vi "DNP3_Master_Station_Main.vi"() -> ()   [LabVIEW 2016, in "DNP3_Master_Station_Template.lvlib"]
uses:
  DNP3_Master_Station_Template.lvlib
  <vilib>/DNP3/DNP3_Master/Operation Mode.ctl
  <vilib>/DNP3/DNP3_Master/Poll Binary Input Variation.ctl
  <vilib>/DNP3/DNP3_Master/Analog Variation.ctl
  <vilib>/DNP3/DNP3_Master/Poll Analog Input Variation.ctl
  <vilib>/DNP3/DNP3_Master/Response Type.ctl
  SubVIs/Global_Bin_Out_Mode.vi
  SubVIs/Global_Bin_In_Var.vi
  SubVIs/Global_An_Out_Var.vi
  SubVIs/Global_An_Out_Mode.vi
  SubVIs/Global_An_In_Var.vi
  <vilib>/DNP3/DNP3_Master.lvlib
panel:
  out "POLL OS IND":bool=TRUE
  out "ENABLE MS IND":bool=TRUE
  out "RESET MS IND":bool
  out "STOP IND":bool
  in  "STOP":bool
  in  "MS Presets":T1(tab)
  in  "Disable Binary TX/RX":bool
  in  "LC1_MS_DNP3_Settings":T6={"Binary Out Mode"=6, "Binary In Variation"=0, "Analog Out Variation"=4, "Analog Out Mode"=6, "Analog In Variation"=0} {"Analog In Variation" items=["Default", "32-bit with Flag", "16-bit with Flag", "32-bit without Flag", "16-bit without Flag", "Single-prec with Flag", "Double-prec with Flag"]; "Analog Out Mode" items=["SBO"=0, "Select"=3, "Operate"=4, "Direct"=5, "Direct No Ack"=6]; "Analog Out Variation" items=["32-bit"=1, "16-bit"=2, "Single-prec"=3, "Double-prec"=4]; "Binary In Variation" items=["Default", "Packed Format", "With Flags"]; "Binary Out Mode" items=["SBO"=0, "Select"=3, "Operate"=4, "Direct"=5, "Direct No Ack"=6]}
  in  "LC1_MS_Network_Settings":T7={"Outstation IP"="10.158.130.104", "DNP3 Port"=20000, "DNP3 Master Address"=30026, "DNP3 Outstation Address"=30024}
  in  "LC1_MS_Network_Settings 2":T7
  in  "LC1_MS_DNP3_Settings 2":T6={"Binary Out Mode"=6, "Binary In Variation"=0, "Analog Out Variation"=4, "Analog Out Mode"=6, "Analog In Variation"=6} {"Analog In Variation" items=["Default", "32-bit with Flag", "16-bit with Flag", "32-bit without Flag", "16-bit without Flag", "Single-prec with Flag", "Double-prec with Flag"]; "Analog Out Mode" items=["SBO"=0, "Select"=3, "Operate"=4, "Direct"=5, "Direct No Ack"=6]; "Analog Out Variation" items=["32-bit"=1, "16-bit"=2, "Single-prec"=3, "Double-prec"=4]; "Binary In Variation" items=["Default", "Packed Format", "With Flags"]; "Binary Out Mode" items=["SBO"=0, "Select"=3, "Operate"=4, "Direct"=5, "Direct No Ack"=6]}
  in  "Disable Binary TX/RX 2":bool
  in  "LC1_MS_Network_Settings 3":T7
  in  "Disable Binary TX/RX 3":bool
  in  "LC1_MS_DNP3_Settings 3":T6={"Binary Out Mode"=6, "Binary In Variation"=0, "Analog Out Variation"=4, "Analog Out Mode"=6, "Analog In Variation"=6} {"Analog In Variation" items=["Default", "32-bit with Flag", "16-bit with Flag", "32-bit without Flag", "16-bit without Flag", "Single-prec with Flag", "Double-prec with Flag"]; "Analog Out Mode" items=["SBO"=0, "Select"=3, "Operate"=4, "Direct"=5, "Direct No Ack"=6]; "Analog Out Variation" items=["32-bit"=1, "16-bit"=2, "Single-prec"=3, "Double-prec"=4]; "Binary In Variation" items=["Default", "Packed Format", "With Flags"]; "Binary Out Mode" items=["SBO"=0, "Select"=3, "Operate"=4, "Direct"=5, "Direct No Ack"=6]}
  out "LC1_MS_RX_Status_Analog":T8=enum."Timeout"
  out "LC1_MS_RX_Status_Binary":T8=enum."Timeout"
  out "LC1_MS_TX_Status_Analog":T8=enum."Success"
  out "LC1_MS_TX_Status_Binary":T8=enum."Cancel"
  out "Main VI Iterations":i32=392
  out "MS SETTINGS CHANGED":bool
  in  "RESET MS":bool caption="Reset Outstation"
  in  "ENABLE MS":bool=TRUE
  in  "POLL OS":bool=TRUE
  out "MS SubVI Iterations":i32=64
  # "Settings Changed; Reset to Update"
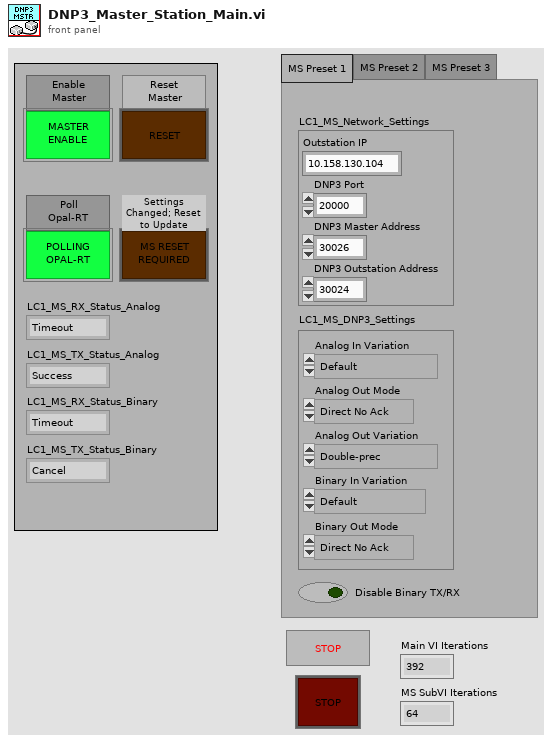
[diagram p1: front panel]
types:
  T1 = enum32{"MS Preset 1", "MS Preset 2", "MS Preset 3"}
  T2 = typedef "DNP3_Master.lvlib/Operation Mode.ctl" = u8
  T3 = typedef "DNP3_Master.lvlib/Poll Binary Input Variation.ctl" = u8
  T4 = typedef "DNP3_Master.lvlib/Analog Variation.ctl" = u8
  T5 = typedef "DNP3_Master.lvlib/Poll Analog Input Variation.ctl" = u8
  T6 = cluster{"Binary Out Mode":T2, "Binary In Variation":T3, "Analog Out Variation":T4, "Analog Out Mode":T2, "Analog In Variation":T5}
  T7 = cluster{"Outstation IP":string, "DNP3 Port":u16, "DNP3 Master Address":u16, "DNP3 Outstation Address":u16}
  T8 = typedef "DNP3_Master.lvlib/Response Type.ctl" = enum16{"Idle", "Buffering", "Pending", "Success", "Failure", "Mismatch", "Status Code", "IIN", "Timeout", "Cancel"}
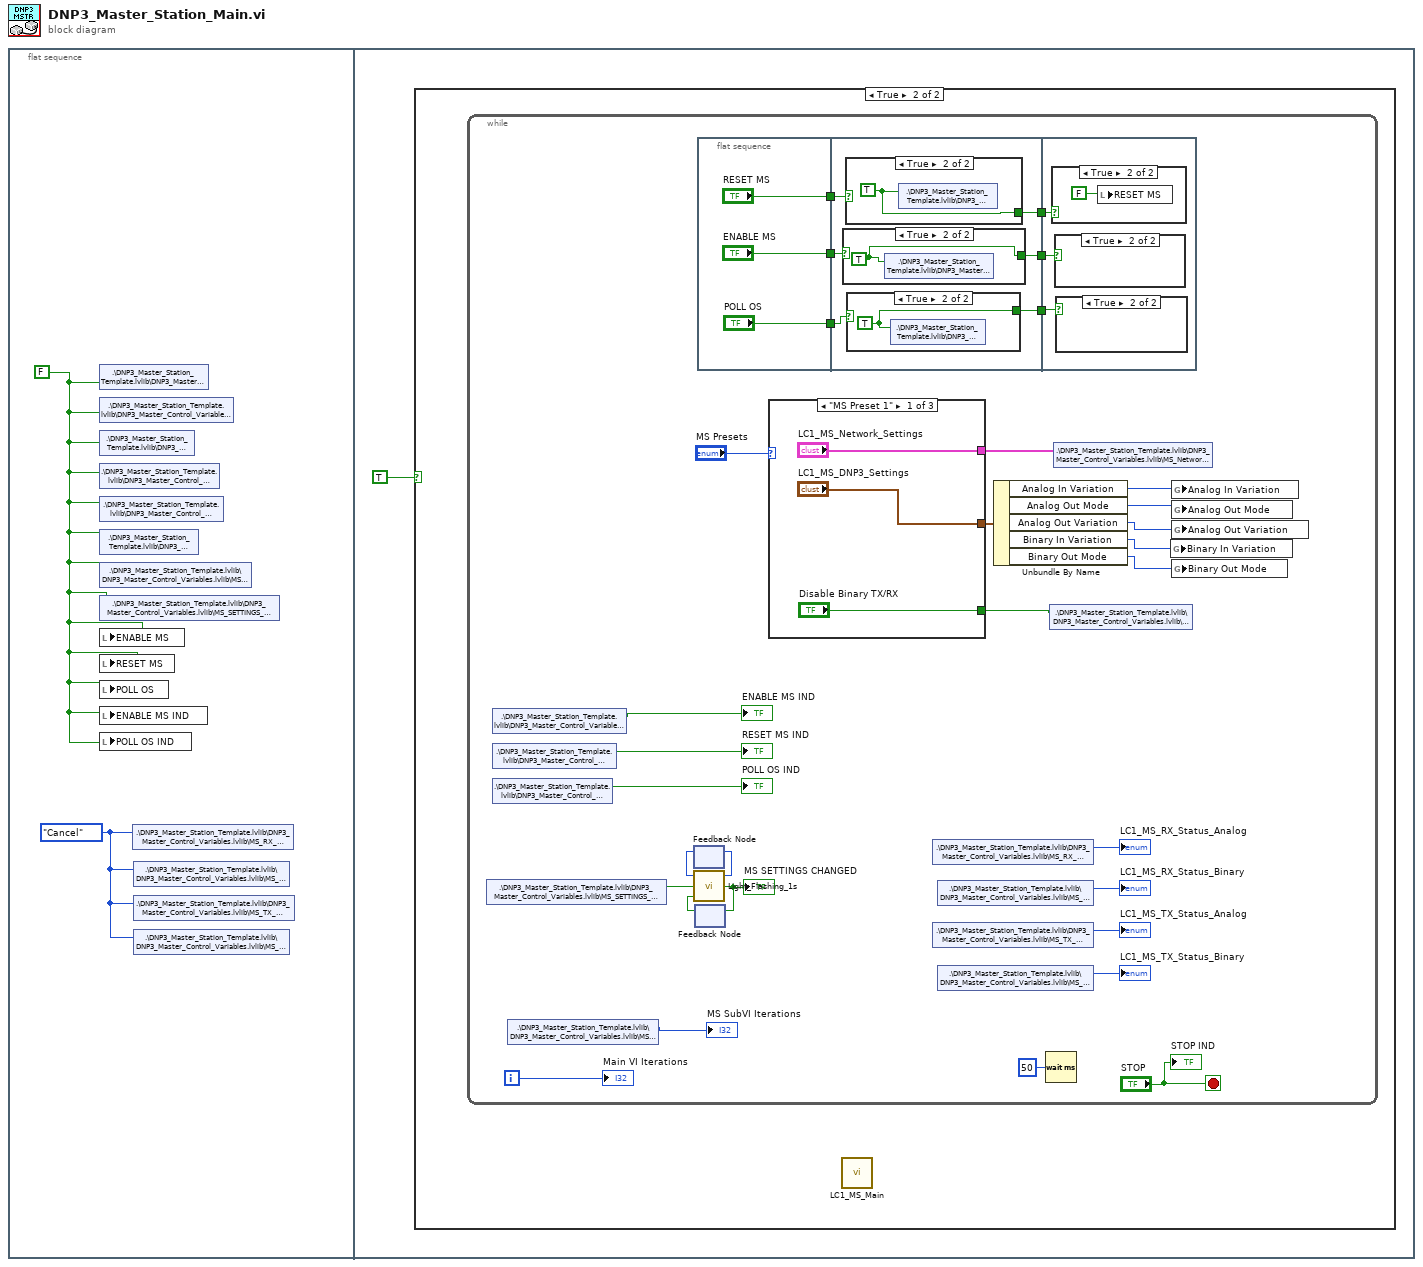
[diagram p0: block diagram]
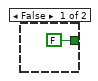
[diagram p3: hidden frame]
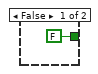
[diagram p4: hidden frame]
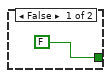
[diagram p5: hidden frame]
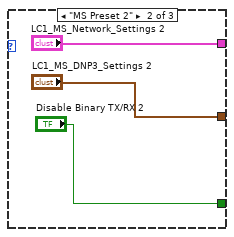
[diagram p9: hidden frame]
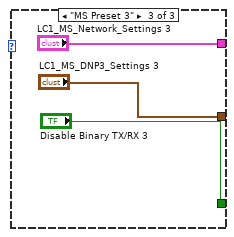
[diagram p10: hidden frame]
diagram:
  n1 = flat-sequence {
    frame #0 {
      w1 = Response_Type."Cancel" ("LC1_MS_RX_Status_Analog")
      w2 = FALSE ("LC1_MS_Enable")
      n2 = shared-variable ".\\DNP3_Master_Station_Template.lvlib\\DNP3_Master_Control_Variables.lvlib\\MS_ENABLE"(w2) -> ()  [unwired: 1 in, 1 out]
      n3 = shared-variable ".\\DNP3_Master_Station_Template.lvlib\\DNP3_Master_Control_Variables.lvlib\\MS_ENABLE_IND"(w2) -> ()  [unwired: 1 in, 1 out]
      n4 = shared-variable ".\\DNP3_Master_Station_Template.lvlib\\DNP3_Master_Control_Variables.lvlib\\MS_POLL"(w2) -> ()  [unwired: 1 in, 1 out]
      n5 = shared-variable ".\\DNP3_Master_Station_Template.lvlib\\DNP3_Master_Control_Variables.lvlib\\MS_POLL_IND"(w2) -> ()  [unwired: 1 in, 1 out]
      n6 = shared-variable ".\\DNP3_Master_Station_Template.lvlib\\DNP3_Master_Control_Variables.lvlib\\MS_RESET_IND"(w2) -> ()  [unwired: 1 in, 1 out]
      n7 = shared-variable ".\\DNP3_Master_Station_Template.lvlib\\DNP3_Master_Control_Variables.lvlib\\MS_RESET"(w2) -> ()  [unwired: 1 in, 1 out]
      n8 = shared-variable ".\\DNP3_Master_Station_Template.lvlib\\DNP3_Master_Control_Variables.lvlib\\MS_RESET_SUCCESS"(w2) -> ()  [unwired: 1 in, 1 out]
      n9 = shared-variable ".\\DNP3_Master_Station_Template.lvlib\\DNP3_Master_Control_Variables.lvlib\\MS_SETTINGS_CHANGED"(w2) -> ()  [unwired: 1 in, 1 out]
      n10 = local write "ENABLE MS"(w2) -> ()
      n11 = local write "RESET MS"(w2) -> ()
      n12 = local write "POLL OS"(w2) -> ()
      n13 = local write "ENABLE MS IND"(w2) -> ()
      n14 = local write "POLL OS IND"(w2) -> ()
      n15 = shared-variable ".\\DNP3_Master_Station_Template.lvlib\\DNP3_Master_Control_Variables.lvlib\\MS_RX_Status_Analog"(w1) -> ()  [unwired: 1 in, 1 out]
      n16 = shared-variable ".\\DNP3_Master_Station_Template.lvlib\\DNP3_Master_Control_Variables.lvlib\\MS_RX_Status_Binary"(w1) -> ()  [unwired: 1 in, 1 out]
      n17 = shared-variable ".\\DNP3_Master_Station_Template.lvlib\\DNP3_Master_Control_Variables.lvlib\\MS_TX_Status_Analog"(w1) -> ()  [unwired: 1 in, 1 out]
      n18 = shared-variable ".\\DNP3_Master_Station_Template.lvlib\\DNP3_Master_Control_Variables.lvlib\\MS_TX_Status_Binary"(w1) -> ()  [unwired: 1 in, 1 out]
    }
    frame #1 {
      n19 = case shown="True" TRUE {
        frame False {
        }
        frame True {
          n20 = while {
            i -> [w31]
            stop <- "STOP" stop-if-true
            n21 = shared-variable ".\\DNP3_Master_Station_Template.lvlib\\DNP3_Master_Control_Variables.lvlib\\MS_SETTINGS_CHANGED"() -> (w15:bool)  [unwired: 1 in, 1 out]
            n22 = shared-variable ".\\DNP3_Master_Station_Template.lvlib\\DNP3_Master_Control_Variables.lvlib\\MS_ENABLE_IND"() -> (→"ENABLE MS IND":bool)  [unwired: 1 in, 1 out]
            n23 = shared-variable ".\\DNP3_Master_Station_Template.lvlib\\DNP3_Master_Control_Variables.lvlib\\MS_RESET_IND"() -> (→"RESET MS IND":bool)  [unwired: 1 in, 1 out]
            n24 = shared-variable ".\\DNP3_Master_Station_Template.lvlib\\DNP3_Master_Control_Variables.lvlib\\MS_POLL_IND"() -> (→"POLL OS IND":bool)  [unwired: 1 in, 1 out]
            n25 = shared-variable ".\\DNP3_Master_Station_Template.lvlib\\DNP3_Master_Control_Variables.lvlib\\MS_SubVI_Iterations"() -> (→"MS SubVI Iterations":i32)  [unwired: 1 in, 1 out]
            n26 = feedback #1() -> (w30:i32)  [unwired: 1 in]
            n27 = feedback #2() -> (w28:bool)  [unwired: 1 in]
            n28 = call "Light_Flashing_1s.vi"("Boolean 3"=w28, "Boolean"=w15, "Numeric 2"=w30) -> ("Boolean 2"=w27:bool, "Numeric"=w29:i32)  [unwired: 1 in]
            "MS SETTINGS CHANGED" <- w27
            n29 = feedback-in #1(w29) -> ()
            n30 = feedback-in #2(w27) -> ()
            n31 = flat-sequence {
              tunnel: ["RESET MS"] -> w26
              tunnel: ["ENABLE MS"] -> w24
              tunnel: ["POLL OS"] -> w22
              tunnel: w26 -> [w43]
              tunnel: [w42] -> w25
              tunnel: w24 -> [w41]
              tunnel: [w40] -> w23
              tunnel: w22 -> [w39]
              tunnel: [w38] -> w21
              tunnel: w25 -> [w52]
              tunnel: w23 -> [w51]
              tunnel: w21 -> [w50]
              frame #0 {
              }
              frame #1 {
                n32 = case shown="True" w41 {
                  tunnel: [FALSE ("LC1_MS_Enable") w47] -> w40
                  frame False {
                  }
                  frame True {
                    w47 = TRUE ("LC1_MS_Enable")
                    n33 = shared-variable ".\\DNP3_Master_Station_Template.lvlib\\DNP3_Master_Control_Variables.lvlib\\MS_ENABLE"(w47) -> ()  [unwired: 1 in, 1 out]
                  }
                }
                n34 = case shown="True" w43 {
                  tunnel: [FALSE ("LC1_MS_Enable") w49] -> w42
                  frame False {
                  }
                  frame True {
                    w49 = TRUE ("LC1_MS_Enable")
                    n35 = shared-variable ".\\DNP3_Master_Station_Template.lvlib\\DNP3_Master_Control_Variables.lvlib\\MS_RESET"(w49) -> ()  [unwired: 1 in, 1 out]
                  }
                }
                n36 = case shown="True" w39 {
                  tunnel: [FALSE ("LC1_MS_Poll") w45] -> w38
                  frame False {
                  }
                  frame True {
                    w45 = TRUE ("LC1_MS_Poll")
                    n37 = shared-variable ".\\DNP3_Master_Station_Template.lvlib\\DNP3_Master_Control_Variables.lvlib\\MS_POLL"(w45) -> ()  [unwired: 1 in, 1 out]
                  }
                }
              }
              frame #2 {
                n38 = case shown="True" w52 {
                  frame False {
                  }
                  frame True {
                    n39 = local write "RESET MS"(FALSE ("ENABLE MS")) -> ()
                  }
                }
                n40 = case shown="True" w51 {
                  frame False {
                  }
                  frame True {
                  }
                }
                n41 = case shown="True" w50 {
                  frame False {
                  }
                  frame True {
                  }
                }
              }
            }
            n42 = case shown="\"MS Preset 1\"" "MS Presets" {
              tunnel: ["LC1_MS_Network_Settings" "LC1_MS_Network_Settings 2" "LC1_MS_Network_Settings 3"] -> w11
              tunnel: ["LC1_MS_DNP3_Settings" "LC1_MS_DNP3_Settings 2" "LC1_MS_DNP3_Settings 3"] -> w9
              tunnel: ["Disable Binary TX/RX" "Disable Binary TX/RX 2" "Disable Binary TX/RX 3"] -> w10
              frame "MS Preset 1" {
              }
              frame "MS Preset 2" {
              }
              frame "MS Preset 3" {
              }
            }
            n43 = shared-variable ".\\DNP3_Master_Station_Template.lvlib\\DNP3_Master_Control_Variables.lvlib\\MS_RX_Status_Analog"() -> (→"LC1_MS_RX_Status_Analog":T8)  [unwired: 1 in, 1 out]
            n44 = shared-variable ".\\DNP3_Master_Station_Template.lvlib\\DNP3_Master_Control_Variables.lvlib\\MS_TX_Status_Analog"() -> (→"LC1_MS_TX_Status_Analog":T8)  [unwired: 1 in, 1 out]
            n45 = shared-variable ".\\DNP3_Master_Station_Template.lvlib\\DNP3_Master_Control_Variables.lvlib\\MS_RX_Status_Binary"() -> (→"LC1_MS_RX_Status_Binary":T8)  [unwired: 1 in, 1 out]
            n46 = shared-variable ".\\DNP3_Master_Station_Template.lvlib\\DNP3_Master_Control_Variables.lvlib\\MS_TX_Status_Binary"() -> (→"LC1_MS_TX_Status_Binary":T8)  [unwired: 1 in, 1 out]
            n47 = Unbundle By Name(w9) -> ("Analog In Variation"=w8:T5, "Analog Out Mode"=w7:T2, "Analog Out Variation"=w6:T4, "Binary In Variation"=w5:T3, "Binary Out Mode"=w4:T2)
            n48 = Wait (ms)(milliseconds to wait=u32 50) -> ()  [unwired: 1 out]
            n49 = shared-variable ".\\DNP3_Master_Station_Template.lvlib\\DNP3_Master_Control_Variables.lvlib\\MS_Disable_Binary"(w10) -> ()  [unwired: 1 in, 1 out]
            n50 = shared-variable ".\\DNP3_Master_Station_Template.lvlib\\DNP3_Master_Control_Variables.lvlib\\MS_Network_Settings"(w11) -> ()  [unwired: 1 in, 1 out]
            n51 = global write "Global_Bin_In_Var.vi" "Binary In Variation"(w5) -> ()
            n52 = global write "Global_An_In_Var.vi" "Analog In Variation"(w8) -> ()
            n53 = global write "Global_An_Out_Mode.vi" "Analog Out Mode"(w7) -> ()
            n54 = global write "Global_An_Out_Var.vi" "Analog Out Variation"(w6) -> ()
            n55 = global write "Global_Bin_Out_Mode.vi" "Binary Out Mode"(w4) -> ()
            "STOP IND" <- "STOP"
            "Main VI Iterations" <- w31
          }
          n56 = call "LC1_MS_Main.vi"() -> ()  [unwired: 12 in]
        }
      }
    }
  }
